vi "Tester.vi"() -> ()   [LabVIEW 2014]
panel:
  out "Voltages":dbl[](array[numeric])=[0.7972994999999994, -0.009129000000000609, -0.009129000000000609, -0.009585900000000258, -0.009129000000000609, -0.009585900000000258, -0.009585900000000258, -0.009585900000000258]
  out "TC Array":dbl[](array[numeric])=[21.380699999999997, 27.4835, 27.4835, 27.4835, 27.4835, 27.378999999999998, 27.4835]
  in  "stop":bool
  out "x-y":u32
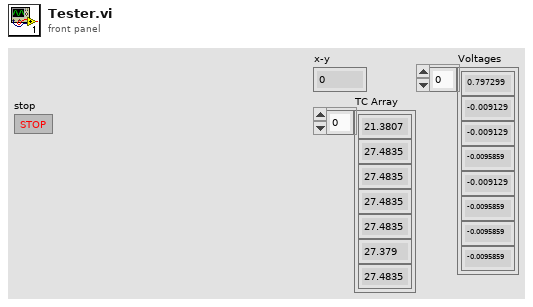
[diagram p1: front panel]
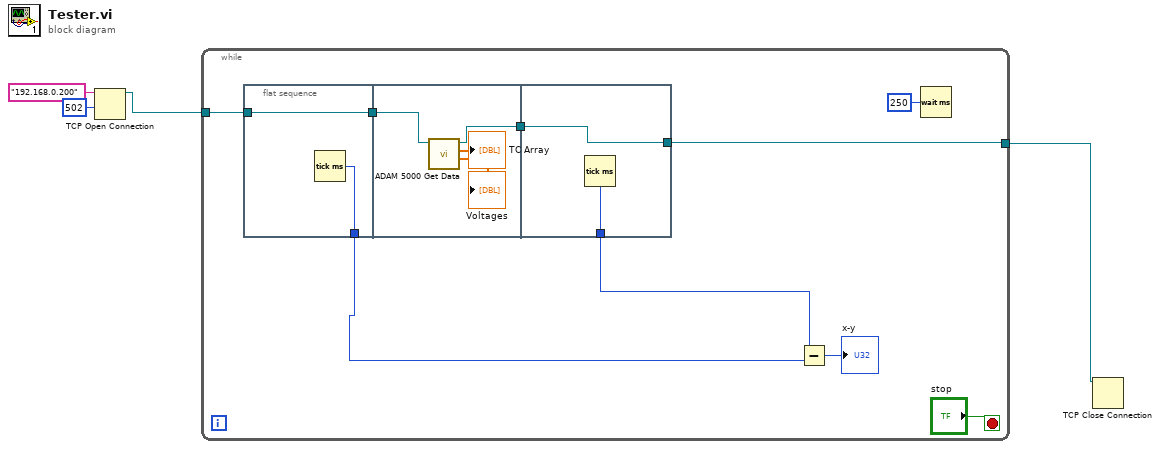
[diagram p0: block diagram]
diagram:
  n1 = TCP Open Connection(address="192.168.0.200", remote port or service name=u16 502) -> (connection ID=w2:refnum<k5>)  [unwired: 3 in, 1 out]
  n2 = while {
    tunnel: w2 -> [w8]
    tunnel: [w5] -> w1
    stop <- "stop" stop-if-true
    n3 = flat-sequence {
      tunnel: [w15] -> w12
      tunnel: w8 -> [w14]
      tunnel: [w14] -> w7
      tunnel: w7 -> [w17]
      tunnel: [w16] -> w6
      tunnel: [w21] -> w13
      tunnel: [w20] -> w5
      tunnel: w6 -> [w20]
      frame #0 {
        n4 = Tick Count (ms)() -> (millisecond timer value=w15:u32)
      }
      frame #1 {
        n5 = call "ADAM 5000 Get Data.vi"("TCP Connection Refnum in"=w17) -> ("Voltages"=→"Voltages":dbl[], "TC Array"=→"TC Array":dbl[], "TCP Connection Refnum (dup)"=w16:refnum<k5>)  [unwired: 8 in]
      }
      frame #2 {
        n6 = Tick Count (ms)() -> (millisecond timer value=w21:u32)
      }
    }
    n7 = Subtract(x=w13, y=w12) -> (x-y=→"x-y":u32)
    n8 = Wait (ms)(milliseconds to wait=u32 250) -> ()  [unwired: 1 out]
  }
  n9 = TCP Close Connection(connection ID=w1) -> ()  [unwired: 2 in, 2 out]
